vi "Update Attributes in Starting.vi"(7 "Attributes in":refnum<class "Attributes.lvclass">, 10 "Transport":refnum<class "Transport.lvclass">) -> (0 "Error out":errorcluster, 5 "Attributes out":refnum<class "Attributes.lvclass">)   [LabVIEW 2025, in "jettl.lvlib"]
uses:
  jettl.lvlib
  Attributes/Attributes/Attributes.lvclass
  Transport/Transport/Transport.lvclass
  Attributes.ctl
  Refs/Refs.lvclass
  Spawn.ctl
  Msg Set.ctl
  Msg/Msg.lvclass
  Actor/Actor.lvclass
  Actor.ctl
  Attributes/Attributes.lvlib
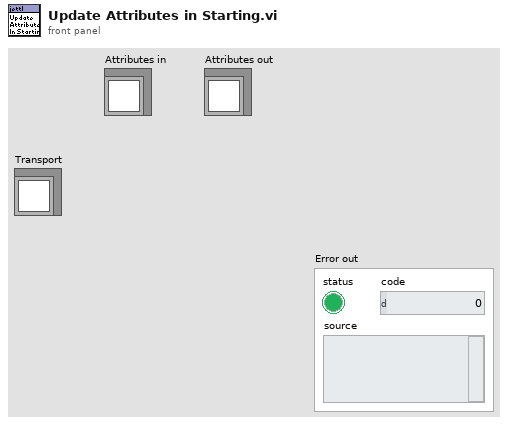
[diagram p1: front panel]
types:
  T1 = typedef "jettl.lvlib/Actor.ctl" = cluster{"Actor Ref":refnum<vi>, "Application Ref":refnum<vi>, "Refs":refnum<class "Refs.lvclass">}
  T2 = typedef "jettl.lvlib/Spawn.ctl" = cluster{"Unified Msg Set":T3, "UID":string, "Parent Attributes":refnum<class "Attributes.lvclass">, "Root":bool, "Persistent Layers":refnum<class "Actor.lvclass">[]}
  T3 = typedef "jettl.lvlib/Msg Set.ctl" = set{refnum<class "Msg.lvclass">}
  T4 = typedef "jettl.lvlib/Attributes.ctl" = cluster{"Spawn":T2, "Actor":T1, "Transport":refnum<class "Transport.lvclass">}
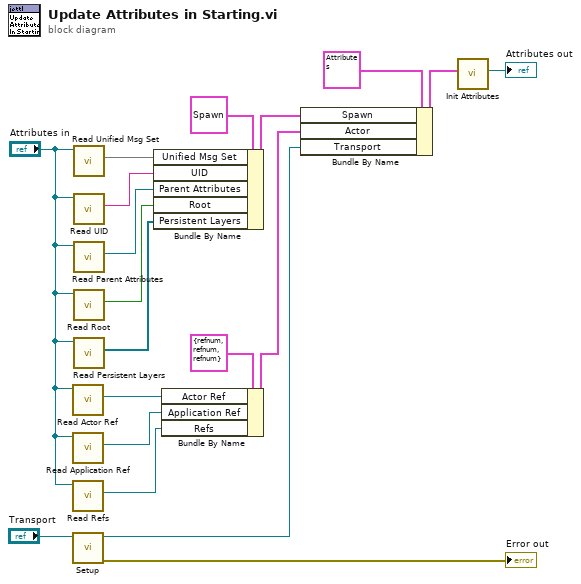
[diagram p0: block diagram]
diagram:
  n1 = call-dynamic "Read Actor Ref.vi"("Attributes in"="Attributes in") -> ("Actor Ref"=w3:refnum<vi>)  [unwired: 10 in]
  n2 = call-dynamic "Read Application Ref.vi"("Attributes in"="Attributes in") -> ("Application Ref"=w2:refnum<vi>)  [unwired: 10 in]
  n3 = call-dynamic "Read Refs.vi"("Attributes in"="Attributes in") -> ("Refs"=w1:refnum<class "Refs.lvclass">)  [unwired: 10 in]
  n4 = call-dynamic "Setup.vi"("Transport in"="Transport") -> ("Error out"=→"Error out":errorcluster, "Transport out"=w6:refnum<class "Transport.lvclass">)  [unwired: 9 in]
  n5 = call-dynamic "Read Unified Msg Set.vi"("Attributes in"="Attributes in") -> ("Unified Msg Set"=w11:T3)  [unwired: 10 in]
  n6 = call-dynamic "Read UID.vi"("Attributes in"="Attributes in") -> ("UID"=w10:string)  [unwired: 10 in]
  n7 = call-dynamic "Read Parent Attributes.vi"("Attributes in"="Attributes in") -> ("Parent Attributes"=w9:refnum<class "Attributes.lvclass">)  [unwired: 10 in]
  n8 = call-dynamic "Read Root.vi"("Attributes in"="Attributes in") -> ("Root"=w8:bool)  [unwired: 10 in]
  n9 = call-dynamic "Read Persistent Layers.vi"("Attributes in"="Attributes in") -> ("Persistent Layers"=w7:refnum<class "Actor.lvclass">[])  [unwired: 10 in]
  n10 = Bundle By Name(cluster=T2 {"Unified Msg Set"={}, "UID"="", "Parent Attributes"=refnum, "Root"=FALSE, "Persistent Layers"=[]} ("Spawn"), "Unified Msg Set"=w11, "UID"=w10, "Parent Attributes"=w9, "Root"=w8, "Persistent Layers"=w7) -> (w12:T2)
  n11 = Bundle By Name(cluster=T1 {"Actor Ref"=refnum, "Application Ref"=refnum, "Refs"=refnum} ("Actor"), "Actor Ref"=w3, "Application Ref"=w2, "Refs"=w1) -> (w4:T1)
  n12 = Bundle By Name(cluster=T4 {"Spawn"={"Unified Msg Set"={}, "UID"="", "Parent Attributes"=refnum, "Root"=FALSE, "Persistent Layers"=[]}, "Actor"={"Actor Ref"=refnum, "Application Ref"=refnum, "Refs"=refnum}, "Transport"=refnum} ("Attributes"), "Spawn"=w12, "Actor"=w4, "Transport"=w6) -> (w17:T4)
  n13 = call "Init Attributes.vi"("Attributes"=w17) -> ("Attributes"=→"Attributes out":refnum<class "Attributes.lvclass">)  [unwired: 10 in]
